vi "SetGlobal.vi"(7 "Numeric":i32) -> ()   [LabVIEW 2019]
uses:
  Global 6.vi
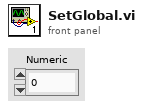
[diagram p1: front panel]
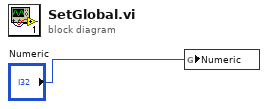
[diagram p0: block diagram]
diagram:
  n1 = global write "Global 6.vi" "Numeric"("Numeric") -> ()
